vi "fifoTesting.vi"() -> ()   [LabVIEW 2016]
uses:
  <vilib>/FPGAPlugInAG/cRIO-9038/niLvFpga_Open_cRIO-9038.vi
  <vilib>/rvi/interface/common/dynamic/niFpgaDynamicAddResources.vi
  <vilib>/FPGAPlugInAG/Dynamic/niLvFpga_Abort_Dynamic.vi
  <vilib>/FPGAPlugInAG/Dynamic/niLvFpga_Reset_Dynamic.vi
  <vilib>/FPGAPlugInAG/Dynamic/niLvFpga_Run_Dynamic.vi
  <vilib>/Utility/error.llb/Error Cluster From Error Code.vi
  <vilib>/rvi/errors/niLvFpgaAdjustHostInterfaceError.vi
  <vilib>/FPGAPlugInAG/Dynamic/niLvFpga_Close_Dynamic.vi
  <vilib>/rvi/interface/nirviOpenFPGA/nirviOpenFPGA.xnode
  FPGA Bitfiles/Modbus_FPGATarget_fifoTesting_0eqS+kh7ysM.lvbitx
  <vilib>/rvi/interface/nirviMethod/nirviMethod.xnode
  <vilib>/rvi/interface/nirviCloseFPGA/nirviCloseFPGA.xnode
  <vilib>/rvi/errors/niLvFpgaMergeErrorWithErrorCode.vi
  <vilib>/FPGAPlugInAG/Dynamic/niLvFpga_WriteFifo_Dynamic.vi
  <vilib>/FPGAPlugInAG/Dynamic/niLvFpga_ReadFifo_Dynamic.vi
panel:
  out "U64Valid":bool
  out "U64Value":u64
  out "U64Time (ms)":u32
  out "U32Valid":bool
  out "U32Value":u32
  out "U32Time (ms)":u32
  out "U16Valid":bool
  out "U16Value":u16
  out "U16Time (ms)":u32
  out "U8Time (ms)":u32
  out "U8Value":u8
  out "U8Valid":bool
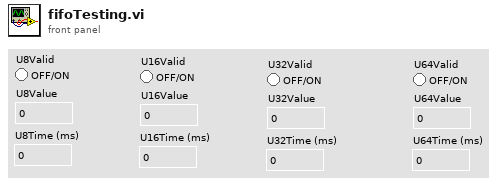
[diagram p1: front panel]
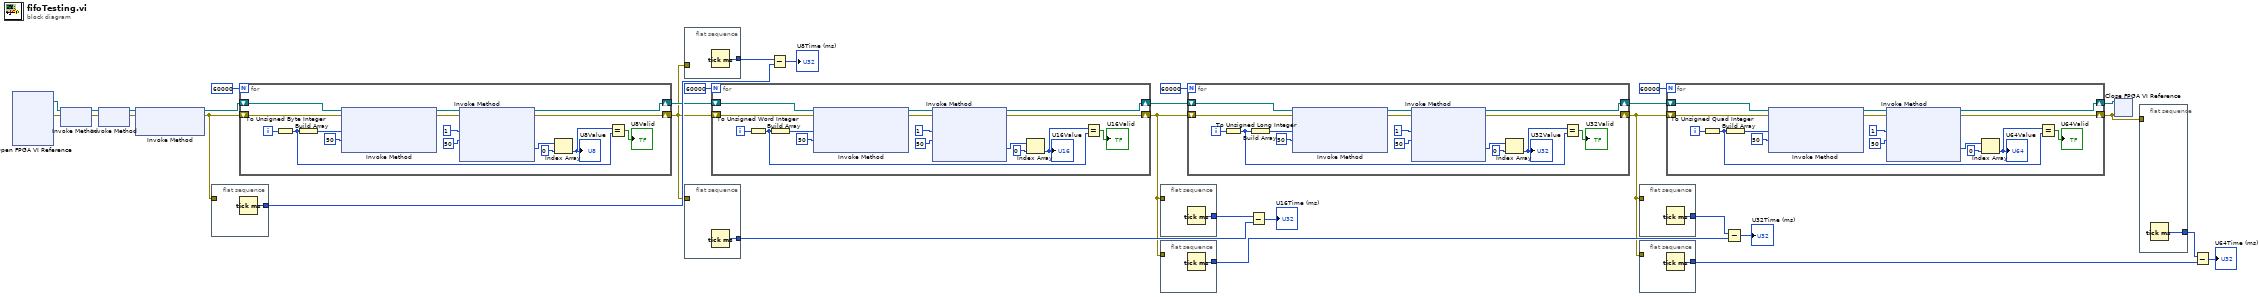
[diagram p0: block diagram]
diagram:
  n1 = xnode "Open FPGA VI Reference"() -> ("FPGA VI Reference Out"=w32:refnum<k20>, "error out"=w27:errorcluster)  [unwired: 2 in]
  n2 = xnode "Invoke Method"("FPGA VI Reference In"=w32, "error in"=w27) -> ("FPGA VI Reference Out"=w31:refnum<k20>, "error out"=w26:errorcluster)
  n3 = xnode "Invoke Method"("FPGA VI Reference In"=w31, "error in"=w26) -> ("FPGA VI Reference Out"=w30:refnum<k20>, "error out"=w25:errorcluster)
  n4 = xnode "Invoke Method"("FPGA VI Reference In"=w30, "error in"=w25) -> ("FPGA VI Reference Out"=w28:refnum<k20>, "error out"=w24:errorcluster)  [unwired: 1 in]
  n5 = flat-sequence {
    tunnel: w24 -> [_]
    tunnel: [w33] -> w22
    frame #0 {
      n6 = Tick Count (ms)() -> (millisecond timer value=w33:u32)
    }
  }
  n7 = for {
    N: 60000 -> [_]
    shift-right: [w43] -> w16
    shift-left: w28 -> [w49]
    shift-right: [w39] -> w15
    shift-left: w24 -> [w41]
    i -> [w48]
    n8 = To Unsigned Byte Integer(number=w48) -> (unsigned 8bit integer=w38:u8)
    n9 = Build Array(w38) -> (w37:u8[])
    n10 = xnode "Invoke Method"("FPGA VI Reference In"=w49, "error in"=w41, "Data"=w37, "Timeout (ms)"=50) -> ("FPGA VI Reference Out"=w46:refnum<k20>, "error out"=w40:errorcluster)  [unwired: 1 out]
    n11 = xnode "Invoke Method"("FPGA VI Reference In"=w46, "error in"=w40, "Number of Elements"=u32 1, "Timeout (ms)"=50) -> ("FPGA VI Reference Out"=w43:refnum<k20>, "error out"=w39:errorcluster, "Data"=w36:u8[])  [unwired: 1 out]
    n12 = Index Array(array=w36, index=0) -> (element=w34:u8)
    "U8Value" <- w34
    n13 = Equal?(x=w34, y=w38) -> (x = y?=→"U8Valid":bool)
  }
  n14 = flat-sequence {
    tunnel: w15 -> [_]
    tunnel: [w50] -> w23
    frame #0 {
      n15 = Tick Count (ms)() -> (millisecond timer value=w50:u32)
    }
  }
  n16 = flat-sequence {
    tunnel: w15 -> [_]
    tunnel: [w51] -> w19
    frame #0 {
      n17 = Tick Count (ms)() -> (millisecond timer value=w51:u32)
    }
  }
  n18 = for {
    N: 60000 -> [_]
    shift-right: [w61] -> w10
    shift-left: w16 -> [w67]
    shift-right: [w57] -> w9
    shift-left: w15 -> [w59]
    i -> [w66]
    n19 = To Unsigned Word Integer(number=w66) -> (unsigned 16bit integer=w56:u16)
    n20 = Build Array(w56) -> (w55:u16[])
    n21 = xnode "Invoke Method"("FPGA VI Reference In"=w67, "error in"=w59, "Data"=w55, "Timeout (ms)"=50) -> ("FPGA VI Reference Out"=w64:refnum<k20>, "error out"=w58:errorcluster)  [unwired: 1 out]
    n22 = xnode "Invoke Method"("FPGA VI Reference In"=w64, "error in"=w58, "Number of Elements"=u32 1, "Timeout (ms)"=50) -> ("FPGA VI Reference Out"=w61:refnum<k20>, "error out"=w57:errorcluster, "Data"=w54:u16[])  [unwired: 1 out]
    n23 = Index Array(array=w54, index=0) -> (element=w52:u16)
    "U16Value" <- w52
    n24 = Equal?(x=w52, y=w56) -> (x = y?=→"U16Valid":bool)
  }
  n25 = Subtract(x=w23, y=w22) -> (x-y=→"U8Time (ms)":u32)
  n26 = flat-sequence {
    tunnel: w9 -> [_]
    tunnel: [w68] -> w18
    frame #0 {
      n27 = Tick Count (ms)() -> (millisecond timer value=w68:u32)
    }
  }
  n28 = flat-sequence {
    tunnel: w9 -> [_]
    tunnel: [w69] -> w12
    frame #0 {
      n29 = Tick Count (ms)() -> (millisecond timer value=w69:u32)
    }
  }
  n30 = for {
    N: 60000 -> [_]
    shift-right: [w79] -> w4
    shift-left: w10 -> [w85]
    shift-right: [w75] -> w3
    shift-left: w9 -> [w77]
    i -> [w84]
    n31 = To Unsigned Long Integer(number=w84) -> (unsigned 32bit integer=w74:u32)
    n32 = Build Array(w74) -> (w73:u32[])
    n33 = xnode "Invoke Method"("FPGA VI Reference In"=w85, "error in"=w77, "Data"=w73, "Timeout (ms)"=50) -> ("FPGA VI Reference Out"=w82:refnum<k20>, "error out"=w76:errorcluster)  [unwired: 1 out]
    n34 = xnode "Invoke Method"("FPGA VI Reference In"=w82, "error in"=w76, "Number of Elements"=u32 1, "Timeout (ms)"=50) -> ("FPGA VI Reference Out"=w79:refnum<k20>, "error out"=w75:errorcluster, "Data"=w72:u32[])  [unwired: 1 out]
    n35 = Index Array(array=w72, index=0) -> (element=w70:u32)
    "U32Value" <- w70
    n36 = Equal?(x=w70, y=w74) -> (x = y?=→"U32Valid":bool)
  }
  n37 = Subtract(x=w18, y=w19) -> (x-y=→"U16Time (ms)":u32)
  n38 = flat-sequence {
    tunnel: w3 -> [_]
    tunnel: [w86] -> w13
    frame #0 {
      n39 = Tick Count (ms)() -> (millisecond timer value=w86:u32)
    }
  }
  n40 = flat-sequence {
    tunnel: w3 -> [_]
    tunnel: [w87] -> w7
    frame #0 {
      n41 = Tick Count (ms)() -> (millisecond timer value=w87:u32)
    }
  }
  n42 = for {
    N: 60000 -> [_]
    shift-right: [w97] -> w2
    shift-left: w4 -> [w103]
    shift-right: [w93] -> w1
    shift-left: w3 -> [w95]
    i -> [w102]
    n43 = To Unsigned Quad Integer(1:w102) -> (0:w92:u64)
    n44 = Build Array(w92) -> (w91:u64[])
    n45 = xnode "Invoke Method"("FPGA VI Reference In"=w103, "error in"=w95, "Data"=w91, "Timeout (ms)"=50) -> ("FPGA VI Reference Out"=w100:refnum<k20>, "error out"=w94:errorcluster)  [unwired: 1 out]
    n46 = xnode "Invoke Method"("FPGA VI Reference In"=w100, "error in"=w94, "Number of Elements"=u32 1, "Timeout (ms)"=50) -> ("FPGA VI Reference Out"=w97:refnum<k20>, "error out"=w93:errorcluster, "Data"=w90:u64[])  [unwired: 1 out]
    n47 = Index Array(array=w90, index=0) -> (element=w88:u64)
    "U64Value" <- w88
    n48 = Equal?(x=w88, y=w92) -> (x = y?=→"U64Valid":bool)
  }
  n49 = Subtract(x=w13, y=w12) -> (x-y=→"U32Time (ms)":u32)
  n50 = xnode "Close FPGA VI Reference"("FPGA VI Reference In"=w2, "error in"=w1) -> ()  [unwired: 1 out]
  n51 = flat-sequence {
    tunnel: w1 -> [_]
    tunnel: [w104] -> w6
    frame #0 {
      n52 = Tick Count (ms)() -> (millisecond timer value=w104:u32)
    }
  }
  n53 = Subtract(x=w6, y=w7) -> (x-y=→"U64Time (ms)":u32)
